vi "SubPnl Size Change.vi"(8 "에러 입력(에러 없음)":errorcluster, 10 "서브 패널":refnum<vi>, 11 "TabControl 입력":refnum<vi>) -> (0 "에러 출력":errorcluster)   [LabVIEW 2020]
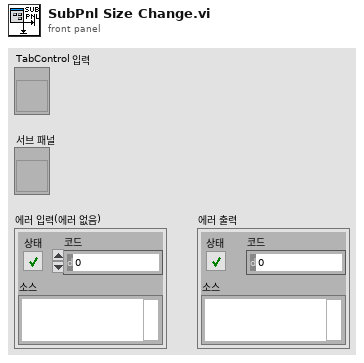
[diagram p1: front panel]
types:
  T1 = typedef "LVBoundsTypeDef.ctl" = cluster{"Width":u32, "Height":u32}
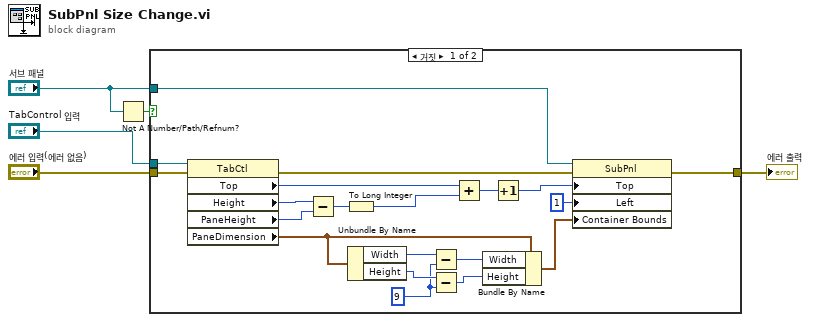
[diagram p0: block diagram]
diagram:
  n1 = Not A Number/Path/Refnum?(number/path/refnum="서브 패널") -> (NaN/Path/Refnum?=w5:bool)
  n2 = case shown="거짓" w5 {
    tunnel: "에러 입력(에러 없음)" -> [w25 w26]
    tunnel: [w23 w26] -> w3
    tunnel: "서브 패널" -> [w20 _]
    tunnel: "TabControl 입력" -> [w19 _]
    frame False {
      w13 = u32 9 ("y")
      n3 = property on="프로퍼티 노드" class="TabCtl"(reference=w19, error in=w25) -> (error out=w24:errorcluster, "Top"=w7:i32, "Height"=w9:u32, "PaneHeight"=w21:u32, "PaneDimension"=w17:T1)  [unwired: 1 out]
      n4 = Subtract(x=w9, y=w21) -> (x-y=w22:u32)
      n5 = To Long Integer(number=w22) -> (32bit integer=w8:i32)
      n6 = Unbundle By Name(w17) -> ("Width"=w15:u32, "Height"=w14:u32)
      n7 = Subtract(x=w15, y=w13) -> (x-y=w12:u32)
      n8 = Subtract(x=w14, y=w13) -> (x-y=w11:u32)
      n9 = Add(x=w7, y=w8) -> (x+y=w18:i32)
      n10 = Bundle By Name(cluster=w17, "Width"=w12, "Height"=w11) -> (w16:T1)
      n11 = Increment(x=w18) -> (x+1=w6:i32)
      n12 = property class="SubPnl"(reference=w20, error in=w24, "Top"=w6, "Left"=1 ("위치:왼쪽"), "Container Bounds"=w16) -> (error out=w23:errorcluster)  [unwired: 1 out]
    }
    frame True {
    }
  }
  "에러 출력" <- w3
